vi "Configure Session.vi"(8 "error in":errorcluster, 11 "Plugin in":refnum<class "MP750510.lvclass">) -> (0 "error out":errorcluster, 3 "Plugin out":refnum<class "MP750510.lvclass">)   [LabVIEW 2025, in "MP750510.lvlib" / "MP750510.lvclass"]
uses:
  MP750510.lvclass
  C:/Program Files/National Instruments/LabVIEW 2025/vi.lib/FlexLogger/SDK/PluginSDK.lvlibp/PEFClasses/SDK/Plugin/Plugin.lvclass
  MP750510.lvclass/MP750510.ctl
  <vilib>/FlexLogger/SDK/PluginSDK.lvlibp/PEFClasses/SDK/Plugin/ParameterAccess/Read String.vi
  <vilib>/FlexLogger/SDK/PluginSDK.lvlibp/PEFClasses/SDK/Channel/ParameterAccess/Read DBL.vi
  <vilib>/FlexLogger/SDK/PluginSDK.lvlibp/PEFClasses/SDK/Channel/ParameterAccess/Read Enum.vi
  <vilib>/FlexLogger/SDK/PluginSDK.lvlibp/PEFClasses/SDK/Plugin/ParameterAccess/Write String.vi
  <vilib>/FlexLogger/SDK/PluginSDK.lvlibp/PEFClasses/SDK/Plugin/Plugin.lvclass
  <vilib>/FlexLogger/SDK/PluginSDK.lvlibp/PEFClasses/SDK/Channel/Channel.lvclass
  C:/Program Files/National Instruments/LabVIEW 2025/vi.lib/FlexLogger/SDK/PluginSDK.lvlibp/PEFClasses/SDK/Processing Element/Processing Element.lvclass
  C:/Users/Steve/Documents/Git/MP750510_Plugin/FlexLogger/MP750510/MP750510.lvclass
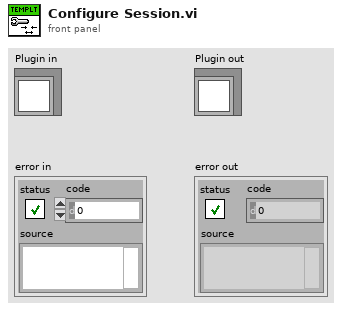
[diagram p1: front panel]
types:
  T1 = cluster{"Freq":dbl, "Amp":dbl, "Offset":dbl, "Phase":dbl, "Wave Type":enum16{"Sine", "Square", "Triangle", "Pulse", "Built In"}, "Initialised":bool}[]
  T2 = cluster{"Freq":dbl, "Amp":dbl, "Offset":dbl, "Phase":dbl, "Wave Type":enum16{"Sine", "Square", "Triangle", "Pulse", "Built In"}, "Initialised":bool}
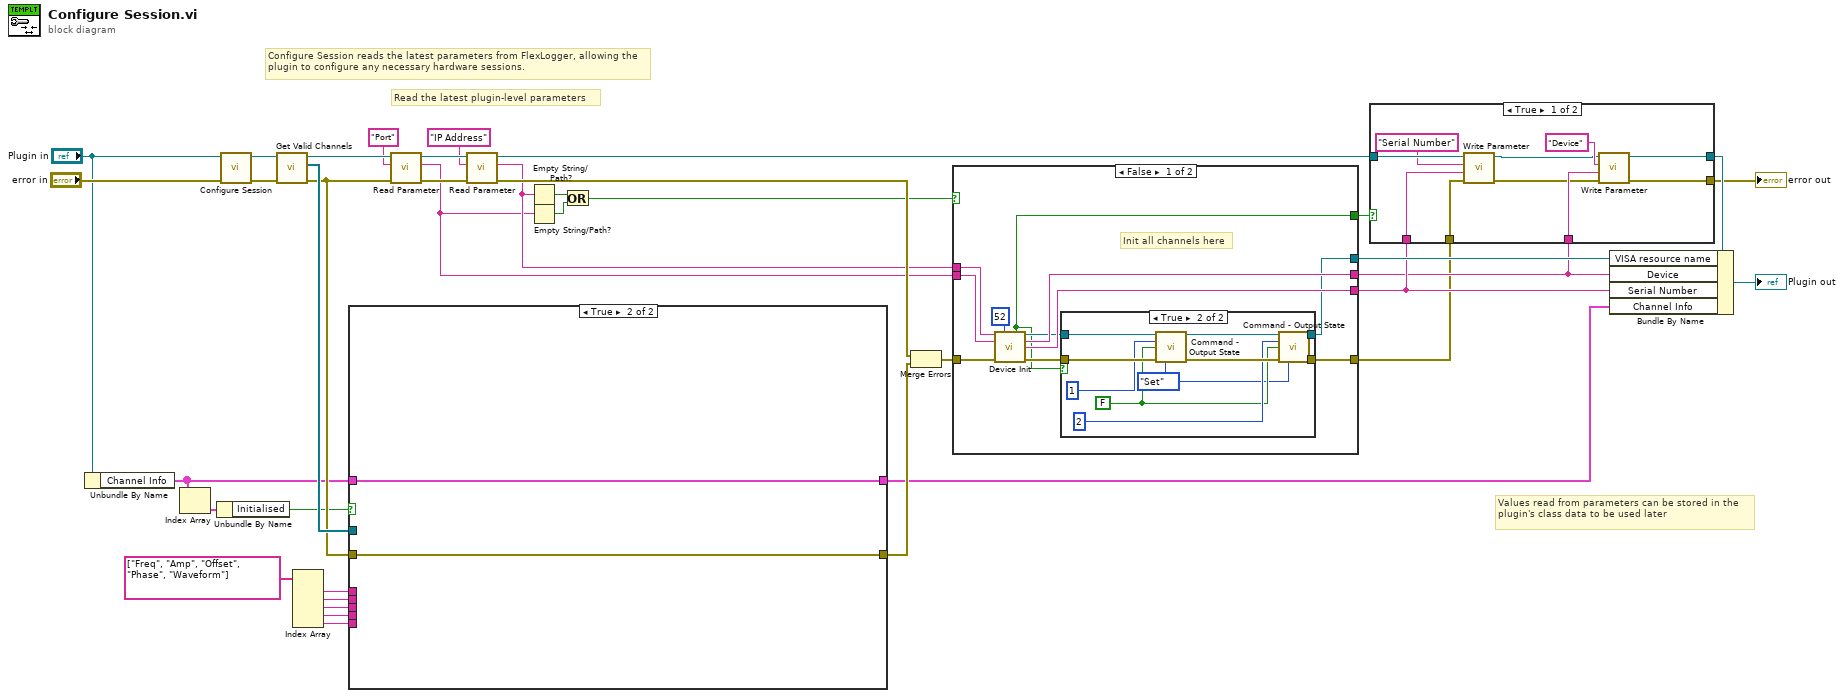
[diagram p0: block diagram]
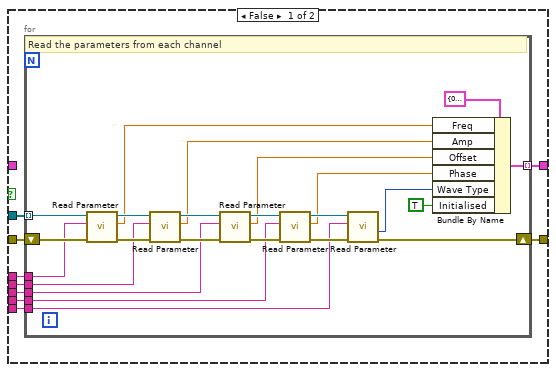
[diagram p2: hidden frame]
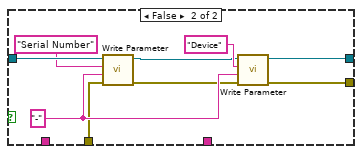
[diagram p3: hidden frame]
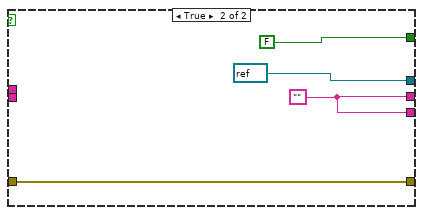
[diagram p5: hidden frame]
diagram:
  # "Read the latest plugin-level parameters"
  # "Configure Session reads the latest parameters from FlexLogger, allowing the plugin to configure any necessary hardware sessions."
  # "Values read from parameters can be stored in the plugin's class data to be used later"
  n1 = Unbundle By Name("Plugin in") -> ("Channel Info"=w1:T1)
  n2 = Index Array(array=w1) -> (element=w3:T2)  [unwired: 1 in]
  n3 = Unbundle By Name(w3) -> ("Initialised"=w2:bool)
  n4 = call-parent "Configure Session.vi"("error in (no error)"="error in", "Processing Element in"="Plugin in") -> ("error out"=w34:errorcluster, "Processing Element out"=w33:refnum<class "MP750510.lvclass">)  [unwired: 8 in]
  n5 = call <vilib>:"Get Valid Channels.vi"("error in (no error)"=w34, "Plugin in"=w33) -> ("error out"=w27:errorcluster, "Channels"=w32:refnum<class "Channel.lvclass">[], "Plugin out"=w31:refnum<class "MP750510.lvclass">)  [unwired: 7 in]
  n6 = Index Array(array=string[] ["Freq", "Amp", "Offset", "Phase", "Waveform"]) -> (element #1=w10:string, element #2=w9:string, element #3=w8:string, element #4=w7:string, element #5=w6:string)  [unwired: 5 in]
  n7 = case shown="True" w2 {
    tunnel: w32 -> [w47 _]
    tunnel: [w46 w72] -> w30
    tunnel: w27 -> [w45 w72]
    tunnel: [w44 w73] -> w5
    tunnel: w10 -> [w43 _]
    tunnel: w9 -> [w42 _]
    tunnel: w8 -> [w41 _]
    tunnel: w7 -> [w40 _]
    tunnel: w6 -> [w39 _]
    tunnel: w1 -> [_ w73]
    frame False {
      n8 = for {
        tunnel: w47 -> [w61] mode=indexing
        shift-right: [w62] -> w46
        shift-left: w45 -> [w63]
        tunnel: [w50] -> w44 mode=indexing
        tunnel: w43 -> [w60]
        tunnel: w42 -> [w59]
        tunnel: w41 -> [w58]
        tunnel: w40 -> [w57]
        tunnel: w39 -> [w56]
        # "Read the parameters from each channel"
        n9 = call-poly <vilib>:"Read Parameter.vi"("error in (no error)"=w63, "Name"=w60, "Channel in"=w61) -> ("error out"=w71:errorcluster, "Value"=w55:dbl, "Channel out"=w67:refnum<class "Channel.lvclass">)  [unwired: 5 in, 1 out]
        n10 = call-poly <vilib>:"Read Parameter.vi"("error in (no error)"=w71, "Name"=w59, "Channel in"=w67) -> ("error out"=w70:errorcluster, "Value"=w54:dbl, "Channel out"=w66:refnum<class "Channel.lvclass">)  [unwired: 5 in, 1 out]
        n11 = call-poly <vilib>:"Read Parameter.vi"("error in (no error)"=w70, "Name"=w58, "Channel in"=w66) -> ("error out"=w69:errorcluster, "Value"=w53:dbl, "Channel out"=w65:refnum<class "Channel.lvclass">)  [unwired: 5 in, 1 out]
        n12 = call-poly <vilib>:"Read Parameter.vi"("error in (no error)"=w69, "Name"=w57, "Channel in"=w65) -> ("error out"=w68:errorcluster, "Value"=w52:dbl, "Channel out"=w64:refnum<class "Channel.lvclass">)  [unwired: 5 in, 1 out]
        n13 = call-poly <vilib>:"Read Parameter.vi"("error in (no error)"=w68, "Name"=w56, "Channel in"=w64) -> ("error out"=w62:errorcluster, "Index"=w51:i32)  [unwired: 4 in, 3 out]
        n14 = Bundle By Name(cluster=T2 {"Freq"=0.0, "Amp"=0.0, "Offset"=0.0, "Phase"=0.0, "Wave Type"=enum."Sine", "Initialised"=FALSE} ("Channel Info"), "Freq"=w55, "Amp"=w54, "Offset"=w53, "Phase"=w52, "Wave Type"=w51, "Initialised"=TRUE) -> (w50:T2)
      }
    }
    frame True {
    }
  }
  n15 = call-poly <vilib>:"Read Parameter.vi"("error in (no error)"=w27, "Name"="Port", "Plugin in"=w31) -> ("error out"=w35:errorcluster, "Value"=w23:string, "Plugin out"=w36:refnum<class "MP750510.lvclass">)  [unwired: 5 in, 1 out]
  n16 = call-poly <vilib>:"Read Parameter.vi"("error in (no error)"=w35, "Name"="IP Address", "Plugin in"=w36) -> ("error out"=w28:errorcluster, "Value"=w24:string, "Plugin out"=w18:refnum<class "MP750510.lvclass">)  [unwired: 5 in, 1 out]
  n17 = Empty String/Path?(string/path=w24) -> (empty?=w21:bool)
  n18 = Empty String/Path?(string/path=w23) -> (empty?=w22:bool)
  n19 = Or(x=w21, y=w22) -> (x .or. y?=w20:bool)
  n20 = Merge Errors(w28, w30) -> (w29:errorcluster)
  n21 = case shown="False" w20 {
    tunnel: [w75 refnum<visa-resource-name> refnum ("VISA resource name")] -> w19
    tunnel: [w77 w98] -> w13
    tunnel: w29 -> [w84 w98]
    tunnel: w24 -> [w83 _]
    tunnel: w23 -> [w82 _]
    tunnel: [w81 w99] -> w14
    tunnel: [w80 w99] -> w15
    tunnel: [w74 FALSE ("Connected?")] -> w16
    frame False {
      # "Init all channels here"
      n22 = call "Device Init.vi"("IP Address"=w83, "Bytes to Read"=u32 52, "Port"=w82, "Error In"=w84) -> ("Connected?"=w74:bool, "VISA resource name"=w76:refnum<visa-resource-name>, "Device"=w81:string, "Serial Number"=w80:string, "Error Out"=w78:errorcluster)  [unwired: 7 in]
      n23 = case shown="True" w74 {
        tunnel: w78 -> [w86 w96]
        tunnel: [w86 w94] -> w77
        tunnel: w76 -> [w85 w93]
        tunnel: [w85 w92] -> w75
        frame False {
        }
        frame True {
          w87 = enum16{"Set", "Get"}."Set" ("Command Type")
          w88 = FALSE ("State")
          n24 = call "Command - Output State.vi"("VISA Refnum in"=w93, "Channel"=1, "State"=w88, "Error In"=w96, "Command Type"=w87) -> ("VISA Refnum out"=w91:refnum<visa-resource-name>, "Error Out"=w95:errorcluster)  [unwired: 8 in, 1 out]
          n25 = call "Command - Output State.vi"("VISA Refnum in"=w91, "Channel"=2, "State"=w88, "Error In"=w95, "Command Type"=w87) -> ("VISA Refnum out"=w92:refnum<visa-resource-name>, "Error Out"=w94:errorcluster)  [unwired: 8 in, 1 out]
        }
      }
    }
    frame True {
      w99 = ""
    }
  }
  n26 = case shown="True" w16 {
    tunnel: w18 -> [w110 w119]
    tunnel: [w101 w111] -> w17
    tunnel: w15 -> [w107 _]
    tunnel: w14 -> [w106 _]
    tunnel: w13 -> [w105 w115]
    tunnel: [w103 w113] -> w12
    frame True {
      n27 = call-poly <vilib>:"Write Parameter.vi"("error in (no error)"=w105, "Value"=w107, "Name"="Serial Number" ("Name (Unique Channel Identifier)"), "Plugin in"=w110) -> ("error out"=w104:errorcluster, "Plugin out"=w102:refnum<class "MP750510.lvclass">)  [unwired: 6 in]
      n28 = call-poly <vilib>:"Write Parameter.vi"("error in (no error)"=w104, "Value"=w106, "Name"="Device" ("Name (Unique Channel Identifier)"), "Plugin in"=w102) -> ("error out"=w103:errorcluster, "Plugin out"=w101:refnum<class "MP750510.lvclass">)  [unwired: 6 in]
    }
    frame False {
      w116 = "-" ("Value")
      n29 = call-poly <vilib>:"Write Parameter.vi"("error in (no error)"=w115, "Value"=w116, "Name"="Serial Number" ("Name (Unique Channel Identifier)"), "Plugin in"=w119) -> ("error out"=w114:errorcluster, "Plugin out"=w112:refnum<class "MP750510.lvclass">)  [unwired: 6 in]
      n30 = call-poly <vilib>:"Write Parameter.vi"("error in (no error)"=w114, "Value"=w116, "Name"="Device" ("Name (Unique Channel Identifier)"), "Plugin in"=w112) -> ("error out"=w113:errorcluster, "Plugin out"=w111:refnum<class "MP750510.lvclass">)  [unwired: 6 in]
    }
  }
  "error out" <- w12
  n31 = Bundle By Name(cluster=w17, "VISA resource name"=w19, "Device"=w14, "Serial Number"=w15, "Channel Info"=w5) -> (→"Plugin out":refnum<class "MP750510.lvclass">)
